vi "bundel_AI_for_Clock_transfer.vi"(9 "FIFO Refs":T1={"FIFO 0"="AI Bundel FIFO 0", "FIFO 1"="AI Bundel FIFO 1", "FIFO 2"="AI Bundel FIFO 2", "FIFO 3"="AI Bundel FIFO 3", "FIFO 4"="AI Bundel FIFO 4", "FIFO 5"="AI Bundel FIFO 5", "FIFO 6"="AI Bundel FIFO 6", "FIFO 7"="AI Bundel FIFO 7"}, 11 "Input Valid":bool) -> (3 "Ready for Input":bool)   [LabVIEW 2014]
uses:
  <vilib>/eio/EIONode/EIONode.xnode
  <vilib>/rvi/eio/common/nirviEmuTemplateMethod_errors.vi
  <vilib>/rvi/DataTransferAndStorage/Container/XNode/niFpgaContainer.xnode
  <vilib>/rvi/FIFO/Fifo_Resource/niFpgaFifoEmulationRefIn.vi
  FPGA_Controls/Acquisition FIFOs Cluster.ctl
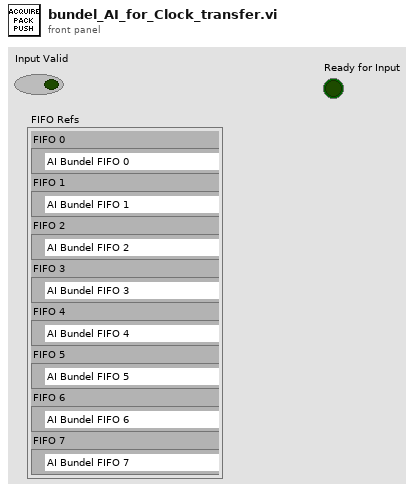
[diagram p1: front panel]
types:
  T1 = typedef "Acquisition FIFOs Cluster.ctl" = cluster{"FIFO 0":refnum<k21>, "FIFO 1":refnum<k21>, "FIFO 2":refnum<k21>, "FIFO 3":refnum<k21>, "FIFO 4":refnum<k21>, "FIFO 5":refnum<k21>, "FIFO 6":refnum<k21>, "FIFO 7":refnum<k21>}
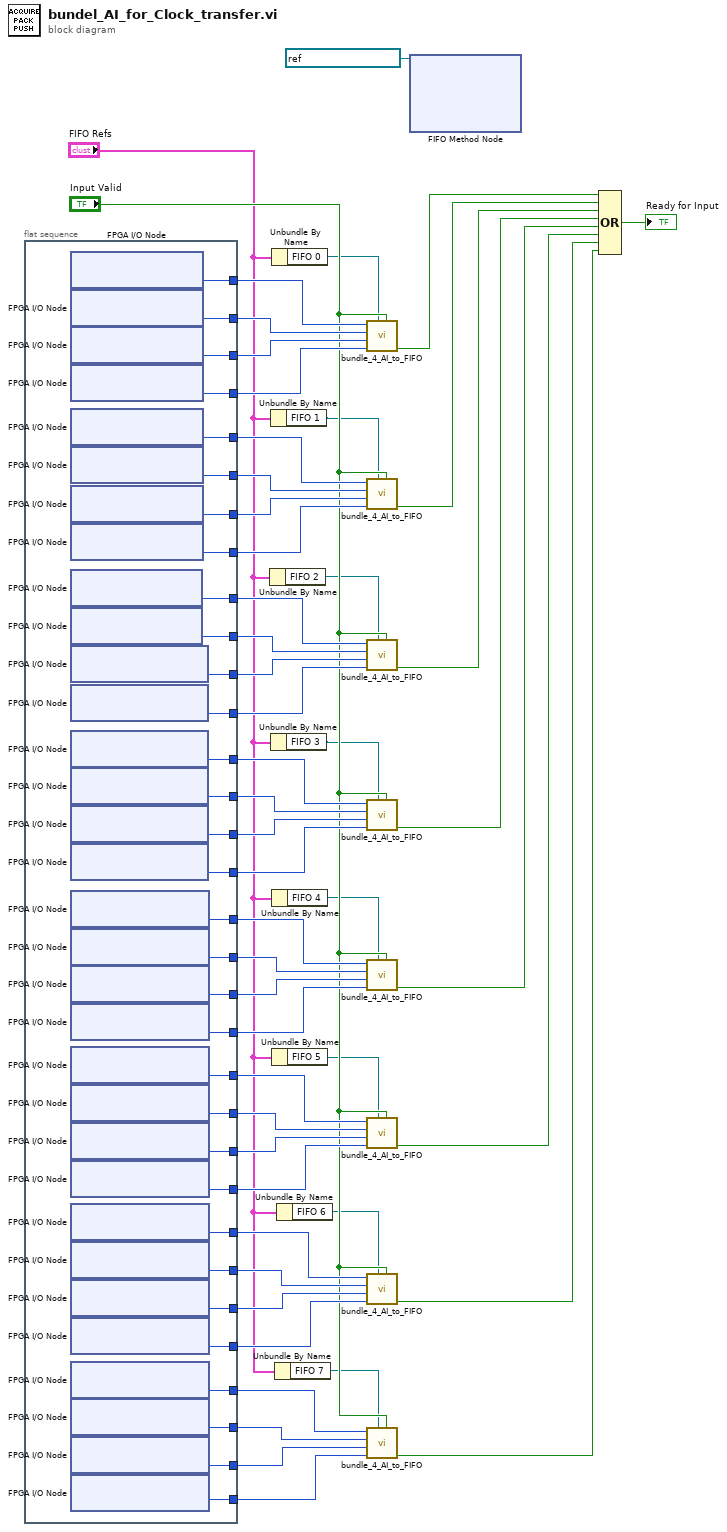
[diagram p0: block diagram]
diagram:
  n1 = flat-sequence {
    tunnel: [w84] -> w51
    tunnel: [w83] -> w50
    tunnel: [w82] -> w49
    tunnel: [w81] -> w48
    tunnel: [w80] -> w47
    tunnel: [w79] -> w46
    tunnel: [w78] -> w45
    tunnel: [w77] -> w44
    tunnel: [w76] -> w43
    tunnel: [w75] -> w42
    tunnel: [w74] -> w41
    tunnel: [w73] -> w40
    tunnel: [w72] -> w39
    tunnel: [w71] -> w37
    tunnel: [w70] -> w36
    tunnel: [w69] -> w38
    tunnel: [w68] -> w20
    tunnel: [w67] -> w21
    tunnel: [w66] -> w22
    tunnel: [w65] -> w23
    tunnel: [w64] -> w26
    tunnel: [w63] -> w24
    tunnel: [w62] -> w25
    tunnel: [w61] -> w27
    tunnel: [w60] -> w28
    tunnel: [w59] -> w29
    tunnel: [w58] -> w30
    tunnel: [w57] -> w31
    tunnel: [w56] -> w32
    tunnel: [w55] -> w33
    tunnel: [w54] -> w34
    tunnel: [w53] -> w35
    frame #0 {
      n2 = xnode "FPGA I/O Node"() -> ("IO Module\\AI A0"=w84:i16)  [unwired: 1 in, 1 out]
      n3 = xnode "FPGA I/O Node"() -> ("IO Module\\AI A1"=w83:i16)  [unwired: 1 in, 1 out]
      n4 = xnode "FPGA I/O Node"() -> ("IO Module\\AI A2"=w82:i16)  [unwired: 1 in, 1 out]
      n5 = xnode "FPGA I/O Node"() -> ("IO Module\\AI A3"=w81:i16)  [unwired: 1 in, 1 out]
      n6 = xnode "FPGA I/O Node"() -> ("IO Module\\AI A4"=w80:i16)  [unwired: 1 in, 1 out]
      n7 = xnode "FPGA I/O Node"() -> ("IO Module\\AI A5"=w79:i16)  [unwired: 1 in, 1 out]
      n8 = xnode "FPGA I/O Node"() -> ("IO Module\\AI A6"=w78:i16)  [unwired: 1 in, 1 out]
      n9 = xnode "FPGA I/O Node"() -> ("IO Module\\AI A7"=w77:i16)  [unwired: 1 in, 1 out]
      n10 = xnode "FPGA I/O Node"() -> ("IO Module\\AI B8"=w76:i16)  [unwired: 1 in, 1 out]
      n11 = xnode "FPGA I/O Node"() -> ("IO Module\\AI B9"=w75:i16)  [unwired: 1 in, 1 out]
      n12 = xnode "FPGA I/O Node"() -> ("IO Module\\AI B10"=w74:i16)  [unwired: 1 in, 1 out]
      n13 = xnode "FPGA I/O Node"() -> ("IO Module\\AI B11"=w73:i16)  [unwired: 1 in, 1 out]
      n14 = xnode "FPGA I/O Node"() -> ("IO Module\\AI B12"=w72:i16)  [unwired: 1 in, 1 out]
      n15 = xnode "FPGA I/O Node"() -> ("IO Module\\AI B13"=w71:i16)  [unwired: 1 in, 1 out]
      n16 = xnode "FPGA I/O Node"() -> ("IO Module\\AI B14"=w70:i16)  [unwired: 1 in, 1 out]
      n17 = xnode "FPGA I/O Node"() -> ("IO Module\\AI B15"=w69:i16)  [unwired: 1 in, 1 out]
      n18 = xnode "FPGA I/O Node"() -> ("IO Module\\AI C16"=w53:i16)  [unwired: 1 in, 1 out]
      n19 = xnode "FPGA I/O Node"() -> ("IO Module\\AI C17"=w54:i16)  [unwired: 1 in, 1 out]
      n20 = xnode "FPGA I/O Node"() -> ("IO Module\\AI C18"=w55:i16)  [unwired: 1 in, 1 out]
      n21 = xnode "FPGA I/O Node"() -> ("IO Module\\AI C19"=w56:i16)  [unwired: 1 in, 1 out]
      n22 = xnode "FPGA I/O Node"() -> ("IO Module\\AI C20"=w57:i16)  [unwired: 1 in, 1 out]
      n23 = xnode "FPGA I/O Node"() -> ("IO Module\\AI C21"=w58:i16)  [unwired: 1 in, 1 out]
      n24 = xnode "FPGA I/O Node"() -> ("IO Module\\AI C22"=w59:i16)  [unwired: 1 in, 1 out]
      n25 = xnode "FPGA I/O Node"() -> ("IO Module\\AI C23"=w60:i16)  [unwired: 1 in, 1 out]
      n26 = xnode "FPGA I/O Node"() -> ("IO Module\\AI D24"=w61:i16)  [unwired: 1 in, 1 out]
      n27 = xnode "FPGA I/O Node"() -> ("IO Module\\AI D25"=w62:i16)  [unwired: 1 in, 1 out]
      n28 = xnode "FPGA I/O Node"() -> ("IO Module\\AI D26"=w63:i16)  [unwired: 1 in, 1 out]
      n29 = xnode "FPGA I/O Node"() -> ("IO Module\\AI D27"=w64:i16)  [unwired: 1 in, 1 out]
      n30 = xnode "FPGA I/O Node"() -> ("IO Module\\AI D28"=w65:i16)  [unwired: 1 in, 1 out]
      n31 = xnode "FPGA I/O Node"() -> ("IO Module\\AI D29"=w66:i16)  [unwired: 1 in, 1 out]
      n32 = xnode "FPGA I/O Node"() -> ("IO Module\\AI D30"=w67:i16)  [unwired: 1 in, 1 out]
      n33 = xnode "FPGA I/O Node"() -> ("IO Module\\AI D31"=w68:i16)  [unwired: 1 in, 1 out]
    }
  }
  n34 = Unbundle By Name("FIFO Refs") -> ("FIFO 2"=w8:refnum<k21>)
  n35 = Unbundle By Name("FIFO Refs") -> ("FIFO 1"=w9:refnum<k21>)
  n36 = Unbundle By Name("FIFO Refs") -> ("FIFO 3"=w7:refnum<k21>)
  n37 = Unbundle By Name("FIFO Refs") -> ("FIFO 0"=w10:refnum<k21>)
  n38 = Unbundle By Name("FIFO Refs") -> ("FIFO 4"=w6:refnum<k21>)
  n39 = Unbundle By Name("FIFO Refs") -> ("FIFO 5"=w3:refnum<k21>)
  n40 = Unbundle By Name("FIFO Refs") -> ("FIFO 7"=w5:refnum<k21>)
  n41 = Unbundle By Name("FIFO Refs") -> ("FIFO 6"=w4:refnum<k21>)
  n42 = call "bundle_4_AI_to_FIFO.vi"("Input Valid"="Input Valid", "FIFO In"=w10, "AI3"=w48, "AI2"=w49, "AI1"=w50, "AI0"=w51) -> ("Ready for Input"=w11:bool)  [unwired: 5 in]
  n43 = call "bundle_4_AI_to_FIFO.vi"("Input Valid"="Input Valid", "FIFO In"=w9, "AI3"=w44, "AI2"=w45, "AI1"=w46, "AI0"=w47) -> ("Ready for Input"=w12:bool)  [unwired: 5 in]
  n44 = call "bundle_4_AI_to_FIFO.vi"("Input Valid"="Input Valid", "FIFO In"=w8, "AI3"=w40, "AI2"=w41, "AI1"=w42, "AI0"=w43) -> ("Ready for Input"=w13:bool)  [unwired: 5 in]
  n45 = call "bundle_4_AI_to_FIFO.vi"("Input Valid"="Input Valid", "FIFO In"=w7, "AI3"=w38, "AI2"=w36, "AI1"=w37, "AI0"=w39) -> ("Ready for Input"=w14:bool)  [unwired: 5 in]
  n46 = call "bundle_4_AI_to_FIFO.vi"("Input Valid"="Input Valid", "FIFO In"=w6, "AI3"=w32, "AI2"=w33, "AI1"=w34, "AI0"=w35) -> ("Ready for Input"=w15:bool)  [unwired: 5 in]
  n47 = call "bundle_4_AI_to_FIFO.vi"("Input Valid"="Input Valid", "FIFO In"=w3, "AI3"=w28, "AI2"=w29, "AI1"=w30, "AI0"=w31) -> ("Ready for Input"=w16:bool)  [unwired: 5 in]
  n48 = call "bundle_4_AI_to_FIFO.vi"("Input Valid"="Input Valid", "FIFO In"=w4, "AI3"=w26, "AI2"=w24, "AI1"=w25, "AI0"=w27) -> ("Ready for Input"=w17:bool)  [unwired: 5 in]
  n49 = call "bundle_4_AI_to_FIFO.vi"("Input Valid"="Input Valid", "FIFO In"=w5, "AI3"=w20, "AI2"=w21, "AI1"=w22, "AI0"=w23) -> ("Ready for Input"=w18:bool)  [unwired: 5 in]
  n50 = xnode ("FIFO Method Node")("FIFO In"=refnum<k21> "AI Bundel FIFO 0") -> ()  [unwired: 2 in, 2 out]
  n51 = Compound Arithmetic op=OR(w11, w12, w13, w14, w15, w16, w17, w18) -> (→"Ready for Input":bool)
